vi "Get ID.vi"(8 "error in (no error)":errorcluster, 11 "Transaction in":refnum<class "Transaction.lvclass">) -> (0 "error out":errorcluster, 2 "ID":i32, 3 "Transaction out":refnum<class "Transaction.lvclass">)   [LabVIEW 2018, in "Transaction.lvclass"]
uses:
  Transaction.lvclass
  Transaction.lvclass/Transaction.ctl
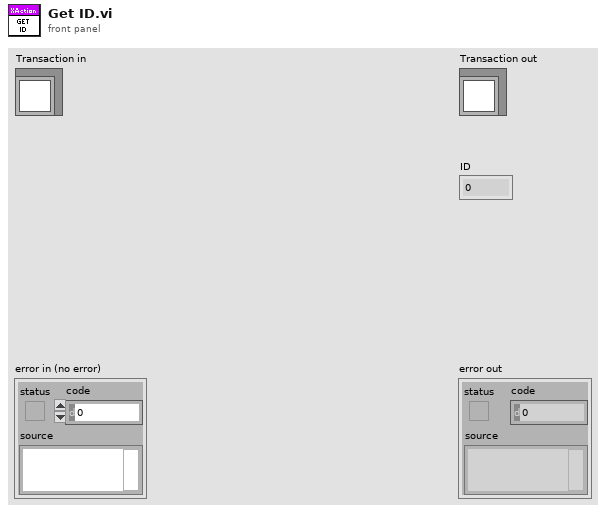
[diagram p1: front panel]
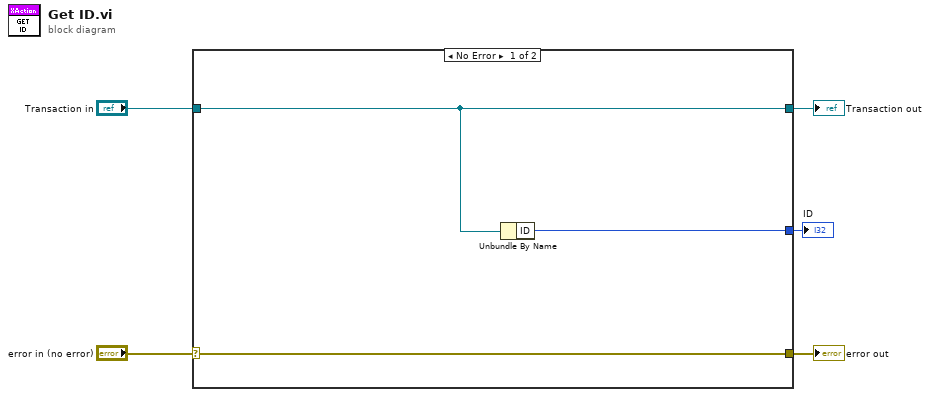
[diagram p0: block diagram]
diagram:
  n1 = case shown="No Error" "error in (no error)" {
    selector: "error in (no error)" -> [w8 w10]
    tunnel: [w8 w10] -> w4
    tunnel: [w7 w9] -> w2
    tunnel: "Transaction in" -> [w7 w9]
    tunnel: [w6 _] -> w1
    frame No Error {
      n2 = Unbundle By Name(w7) -> ("ID"=w6:i32)
    }
    frame Error {
    }
  }
  "error out" <- w4
  "Transaction out" <- w2
  "ID" <- w1
